vi "Order build columns and values array.vi"(10 "Order":T1, 11 "ColunmsList":string[](array[string])) -> (2 "Order values Array":string[](array[string]), 3 "Order Columns Array":string[](array[string]))   [LabVIEW 2015, in "SQLite.lvclass"]
uses:
  SQLite.lvclass
  Order.ctl
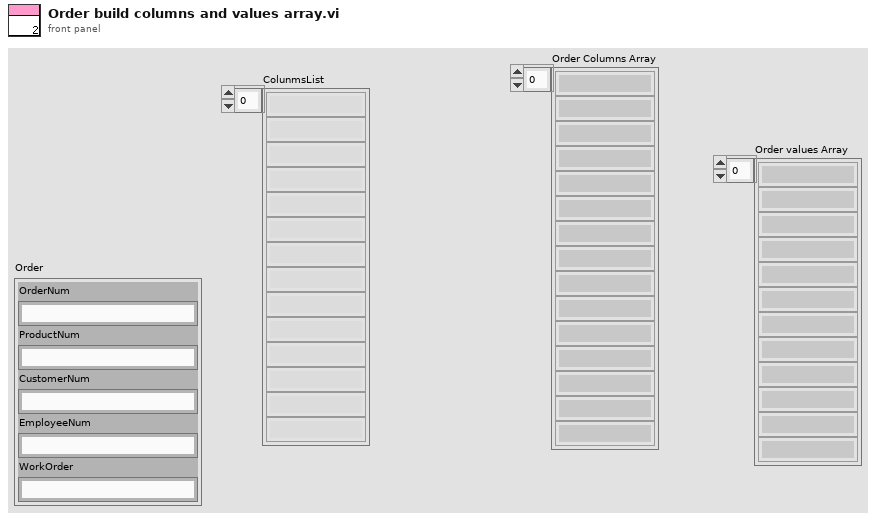
[diagram p1: front panel]
types:
  T1 = typedef "SQLite.lvclass/Order.ctl" = cluster{"OrderNum":string, "ProductNum":string, "CustomerNum":string, "EmployeeNum":string, "WorkOrder":string}
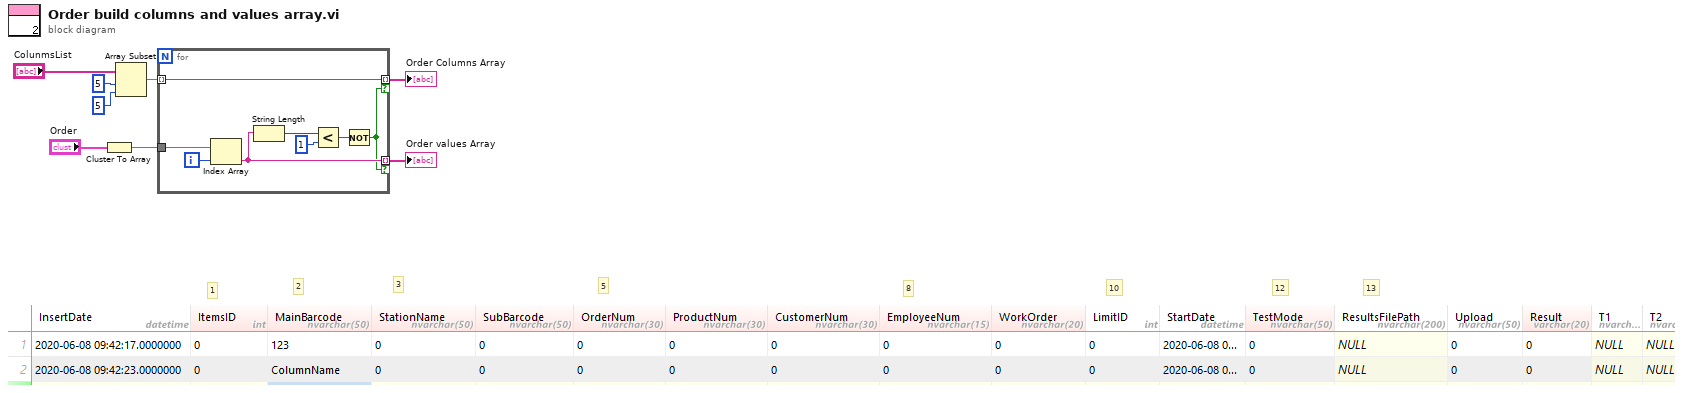
[diagram p0: block diagram]
diagram:
  # "13"
  # "12"
  # "10"
  # "8"
  # "5"
  # "3"
  # "2"
  # "1"
  n1 = Cluster To Array(cluster="Order") -> (array=w3:string[])
  n2 = Array Subset(array="ColunmsList", index=5, length=5) -> (w5:string[])
  n3 = for {
    tunnel: w5 -> [w16] mode=indexing
    tunnel: w3 -> [w13]
    tunnel: [w16] -> w2 mode=indexing if=w9
    tunnel: [w10] -> w1 mode=indexing if=w9
    i -> [w12]
    n4 = Index Array(array=w13, index=w12) -> (element=w10:string)
    n5 = String Length(string=w10) -> (length=w14:i32)
    n6 = Less?(x=w14, y=1) -> (x < y?=w11:bool)
    n7 = Not(x=w11) -> (.not. x?=w9:bool)
  }
  "Order Columns Array" <- w2
  "Order values Array" <- w1
